vi "Configure Correction Characteristic.vi"(8 "error in (no error)":errorcluster, 9 "Correction Name (1: Correction 1)":i32(ring)=1 items=["Correction 1"=1, "Correction 2"=2, "Correction 3"=3, "Correction 4"=4], 10 "Enable Antenna Unit (F: Disable)":bool, 11 "VISA resource name":refnum<visa-resource-name>) -> (0 "error out":errorcluster, 3 "VISA resource name out":refnum<visa-resource-name>)   [LabVIEW 2022 SP3, in "Agilent N934X Series.lvlib"]
doc: "Configure the correction settings.\n\nNote:\nThis VI is only applicable for N9321C, N9322C, N9323C, N9324C models."
uses:
  <instrlib>/Agilent N934X Series/Agilent N934X Series.lvlib
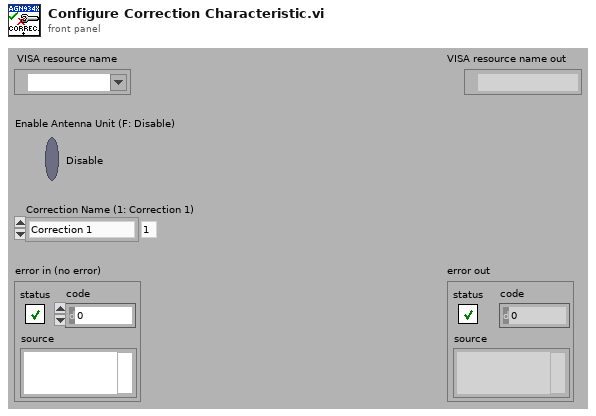
[diagram p1: front panel]
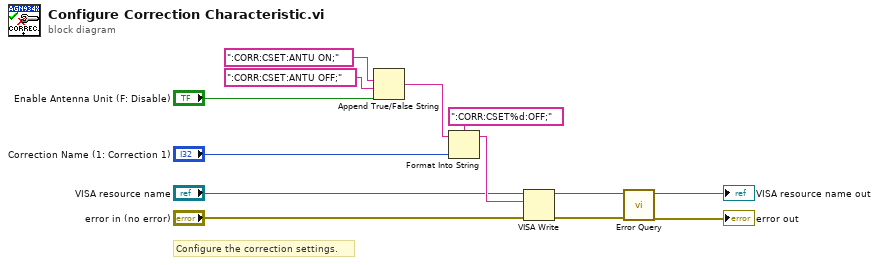
[diagram p0: block diagram]
diagram:
  # "Configure the correction settings."
  n1 = Append True/False String(1:"Enable Antenna Unit (F: Disable)", 2:":CORR:CSET:ANTU OFF;", 3:":CORR:CSET:ANTU ON;") -> (0:w10:string)  [unwired: 1 in]
  n2 = Format Into String(format string=":CORR:CSET%d:OFF;", initial string=w10, "Correction Name (1: Correction 1)") -> (resulting string=w7:string)  [unwired: 1 in, 1 out]
  n3 = VISA Write(VISA resource name="VISA resource name", write buffer=w7, error in (no error)="error in (no error)") -> (VISA resource name out=w4:refnum<visa-resource-name>, error out=w3:errorcluster)  [unwired: 1 out]
  n4 = call <instrlib>:"Error Query.vi"("error in (no error)"=w3, "VISA resource name"=w4) -> ("error out"=→"error out":errorcluster, "VISA resource name out"=→"VISA resource name out":refnum<visa-resource-name>)  [unwired: 6 in, 2 out]
